vi "write_ss_with_header.vi"(0 "temp":dbl[](array[numeric]), 5 "power":dbl[](array[numeric])) -> ()   [LabVIEW 2016]
doc: "Writes a text header and a 2D array to a file from the path output.\n\nThe parser string is [CR, CR, DDD, CR, CR].\n\nMuhannad Alghamdi\nPhysics 350"
uses:
  <vilib>/Utility/file.llb/Write Delimited Spreadsheet (DBL).vi
panel:
  in  "string":string
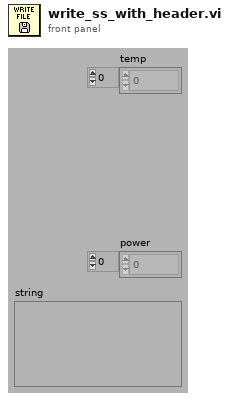
[diagram p1: front panel]
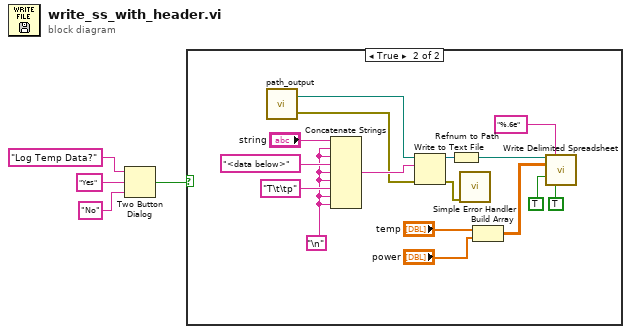
[diagram p0: block diagram]
diagram:
  n1 = Two Button Dialog(message="Log Temp Data?", 1:"No" ("F button name (\"Cancel\")"), 2:"Yes" ("T button name (\"OK\")")) -> (T button?=w4:bool)
  n2 = case shown="True" w4 {
    frame False {
    }
    frame True {
      w5 = "\n"
      n3 = call "path_output.vi"() -> ("Path output"=w8:path, "Error out"=w7:errorcluster)  [unwired: 1 in]
      n4 = Concatenate Strings("string", w5, w5, "<data below>", w5, w5, "T\t\tp" ("string"), w5, w5) -> (w17:string)
      n5 = Write to Text File(file (use dialog)=w8, text=w17, error in=w7) -> (refnum out=w16:refnum<file>, error out=w14:errorcluster)  [unwired: 1 in, 1 out]
      n6 = Refnum to Path(1:w16) -> (0:w15:path)
      n7 = call <vilib>:"Simple Error Handler.vi"("error in (no error)"=w14) -> ()  [unwired: 4 in, 5 out]
      n8 = Build Array("temp", "power") -> (w9:dbl[][])
      n9 = call-poly <vilib>:"Write Delimited Spreadsheet.vi"("file path (dialog if empty)"=w15, "format (%.3f)"="%.6e", "2D data"=w9, "append to file? (new file:F)"=TRUE, "transpose? (no:F)"=TRUE ("Transpose Data?")) -> ()  [unwired: 9 in, 2 out]
    }
  }
